vi "test-math-utils.vi"(8 "error in (no error)":errorcluster) -> (0 "error out":errorcluster, 3 "ALL TESTS PASSED":bool)   [LabVIEW 2019]
uses:
  <vilib>/Rock Robotics/WPI/ThirdParty/JAS_Junk/TrajLib/Trajectory_Library.lvlib
panel:
  out "Test 32":bool
  out "Test 31":bool
  out "Test 30":bool
  out "Test 29":bool
  out "Test 28":bool
  out "Test 27":bool
  out "Test 26":bool
  out "Test 25":bool
  out "mod 24":dbl
  out "Test 24":bool
  out "mod 23":dbl
  out "Test 23":bool
  out "mod 22":dbl
  out "Test 22":bool
  out "mod 21":dbl
  out "Test 21":bool
  out "mod 20":dbl
  out "Test 20":bool
  out "mod 19":dbl
  out "Test 19":bool
  out "mod 18":dbl
  out "mod 17":dbl
  out "mod 16":dbl
  out "Test 18":bool
  out "Test 17":bool
  out "Test 16":bool
  out "Test 15":bool
  out "Test 14":bool
  out "Test 13":bool
  out "Test 12":bool
  out "Test 11":bool
  out "Test 10":bool
  out "Test 9":bool
  out "Test 8":bool
  out "Test 7":bool
  out "Test 6":bool
  out "Test 5":bool
  out "Test 4":bool
  out "Test 3":bool
  out "Test 2":bool
  out "Test 1":bool
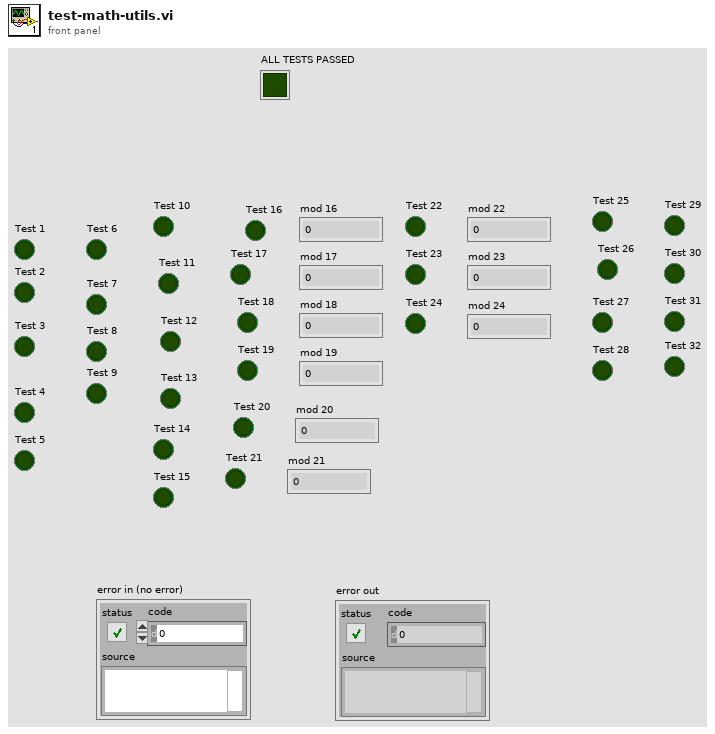
[diagram p1: front panel]
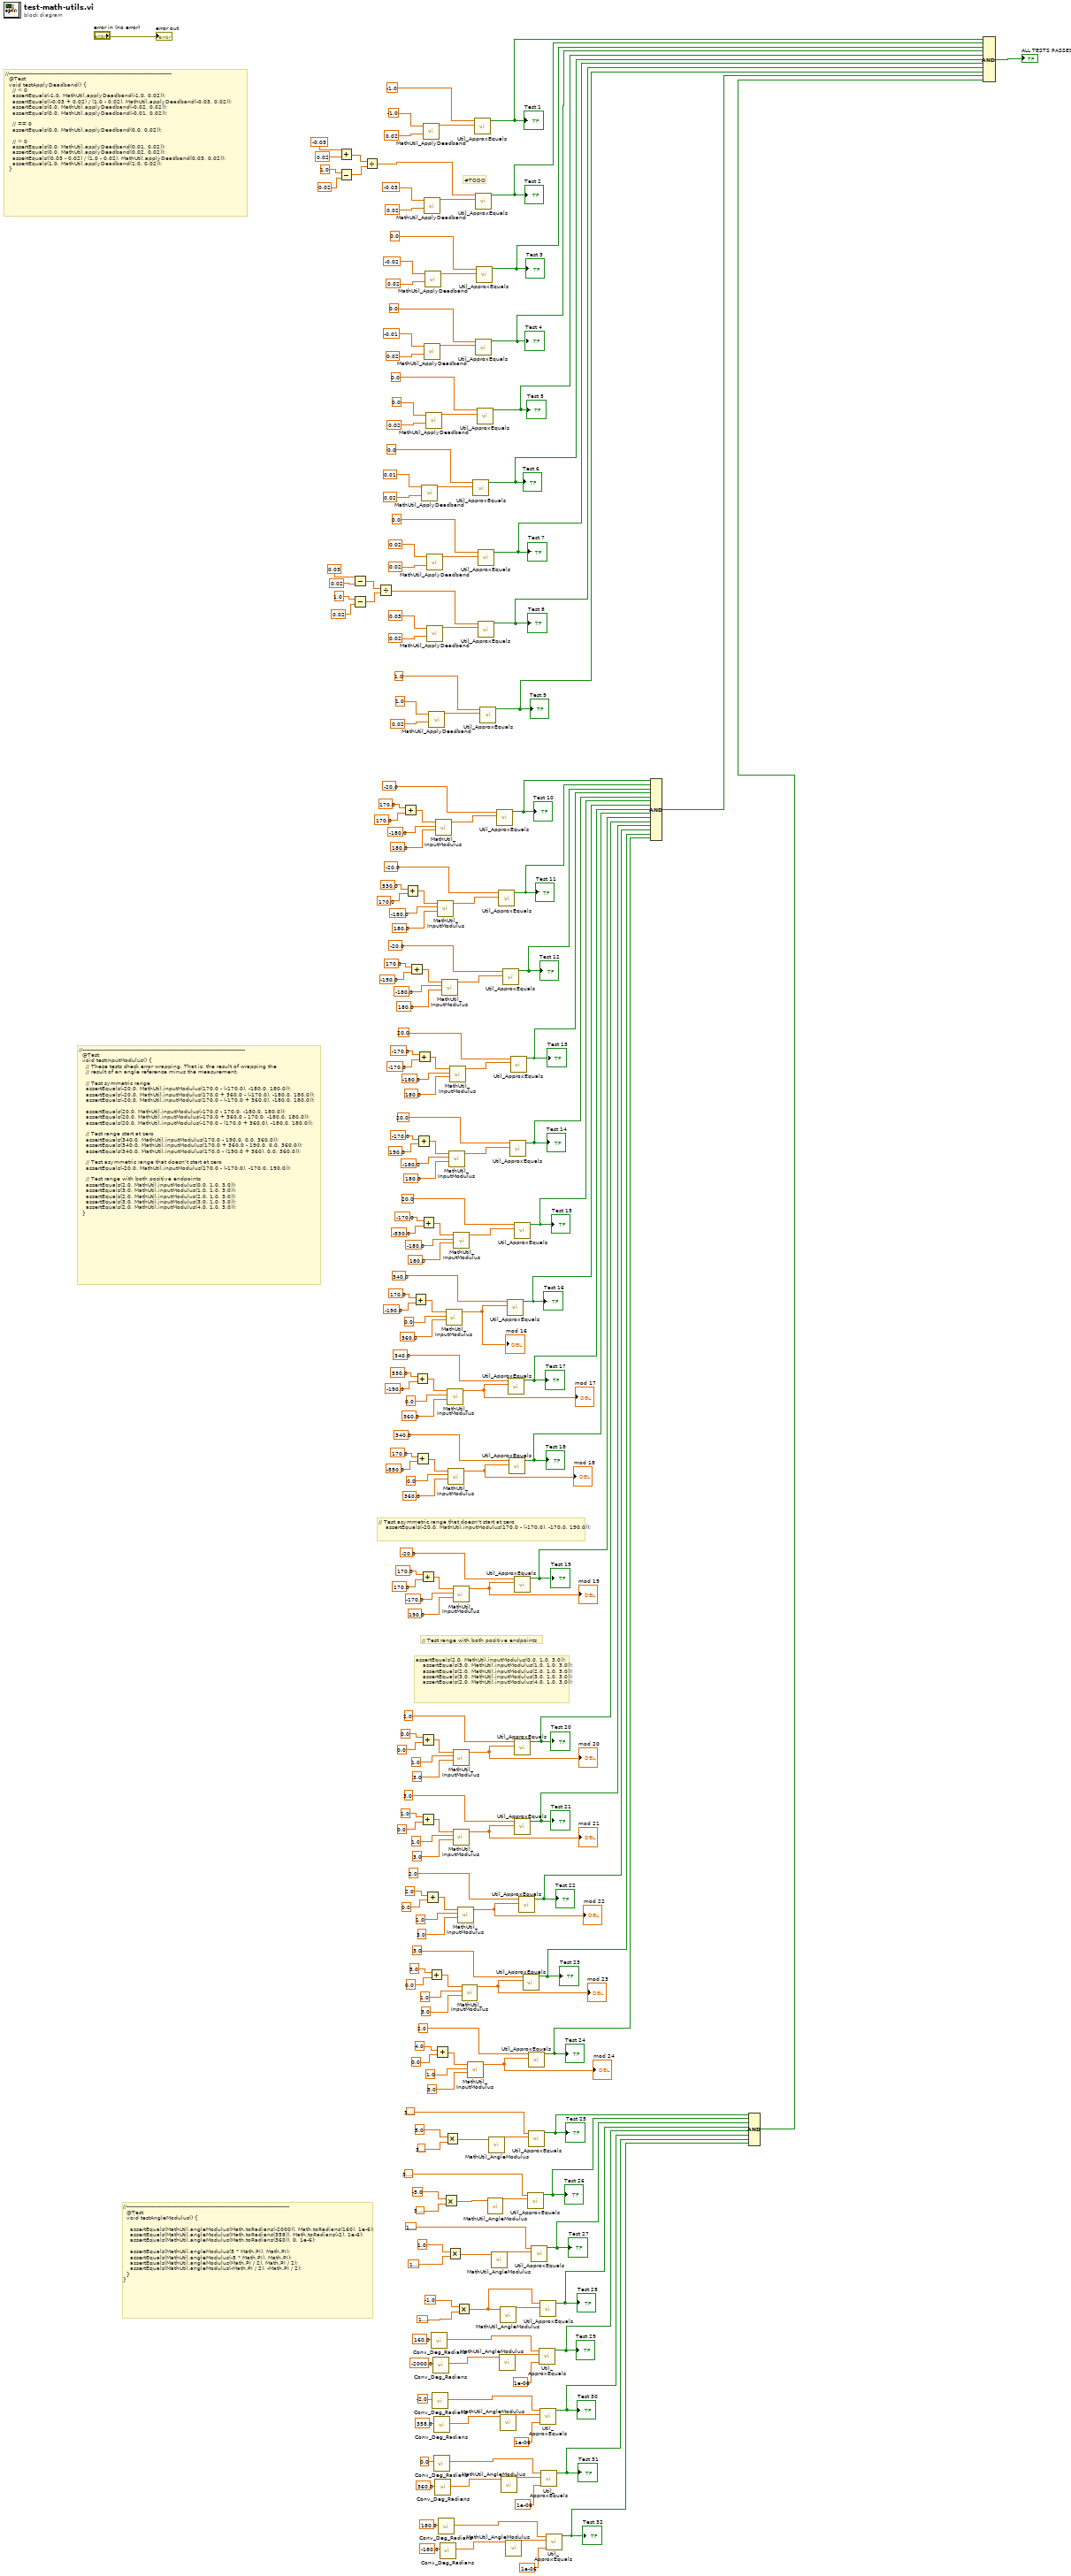
[diagram p0: block diagram]
diagram:
  # "assertEquals(2.0, MathUtil.inputModulus(0.0, 1.0, 3.0));\n    assertEquals(3.0, MathUtil.inputModulus(1.0, 1.0, 3.0));\n    assertEquals(2.0, MathUtil.inputModulus(2.0, 1.0, 3.0));\n    assertEquals(3.0, MathUtil.inputModulus(3.0, 1.0, 3.0));\n    assertEquals(2.0, MathUtil.inputModulus(4.0, 1.0, 3.0));"
  # "// Test range with both positive endpoints"
  # "// Test asymmetric range that doesn't start at zero\n    assertEquals(-20.0, MathUtil.inputModulus(170.0 - (-170.0), -170.0, 190.0));"
  # "#TODO"
  # "//--------------------------------------------------------------------------------------------\n  @Test\n  void testInputModulus() {\n    // These tests check error wrapping. That is, the result of wrapping the\n    // result of an angle reference minus the measurement.\n\n    // Test symmetric range\n    assertEquals(-20.0, MathUtil.inputModulus(170.0 - (-170.0), -180.0, 180.0));\n    assertEquals(-20.0, MathUtil.inputModulus(170.0 + 360.0 - (-170.0), -180.0, 180.0));\n    assertEquals(-20.0, MathUtil.inputModulus(170.0 - (-170.0 + 360.0), -180.0, 180.0));\n\n    assertEquals(20.0, MathUtil.inputModulus(-170.0 - 170.0, -180.0, 180.0));\n    assertEquals(20.0, MathUtil.inputModulus(-170.0 + 360.0 - 170.0, -180.0, 180.0));\n    assertEquals(20.0, MathUtil.inputModulus(-170.0 - (170.0 + 360.0), -180.0, 180.0));\n\n    // Test range start at zero\n    assertEquals(340.0, MathUtil.inputModulus(170.0 - 190.0, 0.0, 360.0));\n    assertEquals(340.0, MathUtil.inputModulus(170.0 + 360.0 - 190.0, 0.0, 360.0));\n    assertEquals(340.0, MathUtil.inputModulus(170.0 - (190.0 + 360), 0.0, 360.0));\n\n    // Test asymmetric range that doesn't start at zero\n    assertEquals(-20.0, MathUtil.inputModulus(170.0 - (-170.0), -170.0, 190.0));\n\n    // Test range with both positive endpoints\n    assertEquals(2.0, MathUtil.inputModulus(0.0, 1.0, 3.0));\n    assertEquals(3.0, MathUtil.inputModulus(1.0, 1.0, 3.0));\n    assertEquals(2.0, MathUtil.inputModulus(2.0, 1.0, 3.0));\n    assertEquals(3.0, MathUtil.inputModulus(3.0, 1.0, 3.0));\n    assertEquals(2.0, MathUtil.inputModulus(4.0, 1.0, 3.0));\n  }"
  # "//--------------------------------------------------------------------------------------------\n  @Test\n  void testApplyDeadband() {\n    // < 0\n    assertEquals(-1.0, MathUtil.applyDeadband(-1.0, 0.02));\n    assertEquals((-0.03 + 0.02) / (1.0 - 0.02), MathUtil.applyDeadband(-0.03, 0.02));\n    assertEquals(0.0, MathUtil.applyDeadband(-0.02, 0.02));\n    assertEquals(0.0, MathUtil.applyDeadband(-0.01, 0.02));\n\n    // == 0\n    assertEquals(0.0, MathUtil.applyDeadband(0.0, 0.02));\n\n    // > 0\n    assertEquals(0.0, MathUtil.applyDeadband(0.01, 0.02));\n    assertEquals(0.0, MathUtil.applyDeadband(0.02, 0.02));\n    assertEquals((0.03 - 0.02) / (1.0 - 0.02), MathUtil.applyDeadband(0.03, 0.02));\n    assertEquals(1.0, MathUtil.applyDeadband(1.0, 0.02));\n  }"
  # "//--------------------------------------------------------------------------------------------\n  @Test\n  void testAngleModulus() {\n\n    assertEquals(MathUtil.angleModulus(Math.toRadians(-2000)), Math.toRadians(160), 1e-6);\n    assertEquals(MathUtil.angleModulus(Math.toRadians(358)), Math.toRadians(-2), 1e-6);\n    assertEquals(MathUtil.angleModulus(Math.toRadians(360)), 0, 1e-6);\n\n    assertEquals(MathUtil.angleModulus(5 * Math.PI), Math.PI);\n    assertEquals(MathUtil.angleModulus(-5 * Math.PI), Math.PI);\n    assertEquals(MathUtil.angleModulus(Math.PI / 2), Math.PI / 2);\n    assertEquals(MathUtil.angleModulus(-Math.PI / 2), -Math.PI / 2);\n  }\n}"
  n1 = Add(x=-0.03, y=0.02) -> (x+y=w187:dbl)
  n2 = Subtract(x=1.0, y=0.02) -> (x-y=w186:dbl)
  n3 = Subtract(x=0.03, y=0.02) -> (x-y=w180:dbl)
  n4 = Subtract(x=1.0, y=0.02) -> (x-y=w179:dbl)
  n5 = Divide(x=w187, y=w186) -> (x/y=w181:dbl)
  n6 = Divide(x=w180, y=w179) -> (x/y=w174:dbl)
  n7 = Add(x=170.0, y=170.0) -> (x+y=w169:dbl)
  n8 = Add(x=530.0, y=170.0) -> (x+y=w162:dbl)
  n9 = Add(x=170.0, y=-190.0) -> (x+y=w155:dbl)
  n10 = Add(x=170.0, y=-190.0) -> (x+y=w127:dbl)
  n11 = Add(x=530.0, y=-190.0) -> (x+y=w120:dbl)
  n12 = Add(x=170.0, y=-550.0) -> (x+y=w113:dbl)
  n13 = Add(x=-170.0, y=190.0) -> (x+y=w141:dbl)
  n14 = Add(x=-170.0, y=-170.0) -> (x+y=w148:dbl)
  n15 = Add(x=170.0, y=170.0) -> (x+y=w106:dbl)
  n16 = Add(x=0.0, y=0.0) -> (x+y=w99:dbl)
  n17 = Add(x=1.0, y=0.0) -> (x+y=w92:dbl)
  n18 = Add(x=-170.0, y=-530.0) -> (x+y=w134:dbl)
  n19 = call <vilib>:"MathUtil_ApplyDeadband.vi"("Deadband"=0.02, "Value"=0.01) -> ("Result"=w211:dbl)  [unwired: 9 in]
  n20 = call <vilib>:"MathUtil_ApplyDeadband.vi"("Deadband"=0.02, "Value"=-1.0) -> ("Result"=w230:dbl)  [unwired: 9 in]
  n21 = call <vilib>:"MathUtil_ApplyDeadband.vi"("Deadband"=0.02, "Value"=-0.03) -> ("Result"=w227:dbl)  [unwired: 9 in]
  n22 = call <vilib>:"MathUtil_ApplyDeadband.vi"("Deadband"=0.02, "Value"=-0.01) -> ("Result"=w219:dbl)  [unwired: 9 in]
  n23 = call <vilib>:"MathUtil_ApplyDeadband.vi"("Deadband"=0.02, "Value"=-0.02) -> ("Result"=w223:dbl)  [unwired: 9 in]
  n24 = Add(x=2.0, y=0.0) -> (x+y=w85:dbl)
  n25 = call <vilib>:"MathUtil_ApplyDeadband.vi"("Deadband"=0.02, "Value"=0.0) -> ("Result"=w215:dbl)  [unwired: 9 in]
  n26 = call <vilib>:"MathUtil_ApplyDeadband.vi"("Deadband"=0.02, "Value"=0.02) -> ("Result"=w207:dbl)  [unwired: 9 in]
  n27 = call <vilib>:"MathUtil_ApplyDeadband.vi"("Deadband"=0.02, "Value"=0.03) -> ("Result"=w204:dbl)  [unwired: 9 in]
  n28 = call <vilib>:"MathUtil_ApplyDeadband.vi"("Deadband"=0.02, "Value"=1.0) -> ("Result"=w200:dbl)  [unwired: 9 in]
  n29 = Add(x=3.0, y=0.0) -> (x+y=w78:dbl)
  n30 = call <vilib>:"Conv_Deg_Radians.vi"("Degress"=160.0) -> ("Radians"=w30:dbl)  [unwired: 10 in]
  n31 = call <vilib>:"Conv_Deg_Radians.vi"("Degress"=-2.0) -> ("Radians"=w24:dbl)  [unwired: 10 in]
  n32 = call <vilib>:"Conv_Deg_Radians.vi"("Degress"=-2000.0) -> ("Radians"=w29:dbl)  [unwired: 10 in]
  n33 = call <vilib>:"Conv_Deg_Radians.vi"("Degress"=0.0) -> ("Radians"=w18:dbl)  [unwired: 10 in]
  n34 = call <vilib>:"Conv_Deg_Radians.vi"("Degress"=358.0) -> ("Radians"=w23:dbl)  [unwired: 10 in]
  n35 = Add(x=4.0, y=0.0) -> (x+y=w71:dbl)
  n36 = call <vilib>:"Conv_Deg_Radians.vi"("Degress"=360.0) -> ("Radians"=w17:dbl)  [unwired: 10 in]
  n37 = call <vilib>:"MathUtil_InputModulus.vi"("Maximum_Input"=180.0, "Minimum_Input"=-180.0, "Input"=w169) -> ("modulus"=w173:dbl)  [unwired: 8 in]
  n38 = call <vilib>:"MathUtil_InputModulus.vi"("Maximum_Input"=180.0, "Minimum_Input"=-180.0, "Input"=w162) -> ("modulus"=w166:dbl)  [unwired: 8 in]
  n39 = call <vilib>:"Conv_Deg_Radians.vi"("Degress"=180.0) -> ("Radians"=w12:dbl)  [unwired: 10 in]
  n40 = call <vilib>:"Conv_Deg_Radians.vi"("Degress"=-180.0) -> ("Radians"=w11:dbl)  [unwired: 10 in]
  n41 = call <vilib>:"MathUtil_InputModulus.vi"("Maximum_Input"=180.0, "Minimum_Input"=-180.0, "Input"=w155) -> ("modulus"=w159:dbl)  [unwired: 8 in]
  n42 = Multiply(x=-5.0, y=3.141592653589793) -> (x*y=w45:dbl)
  n43 = Multiply(x=5.0, y=3.141592653589793) -> (x*y=w50:dbl)
  n44 = call <vilib>:"MathUtil_InputModulus.vi"("Maximum_Input"=360.0, "Minimum_Input"=0.0, "Input"=w127) -> ("modulus"=w131:dbl)  [unwired: 8 in]
  "mod 16" <- w131
  n45 = call <vilib>:"MathUtil_InputModulus.vi"("Maximum_Input"=360.0, "Minimum_Input"=0.0, "Input"=w120) -> ("modulus"=w124:dbl)  [unwired: 8 in]
  "mod 17" <- w124
  n46 = Multiply(x=1.0, y=1.5707963267948966) -> (x*y=w41:dbl)
  n47 = call <vilib>:"MathUtil_InputModulus.vi"("Maximum_Input"=360.0, "Minimum_Input"=0.0, "Input"=w113) -> ("modulus"=w117:dbl)  [unwired: 8 in]
  "mod 18" <- w117
  n48 = call <vilib>:"MathUtil_InputModulus.vi"("Maximum_Input"=180.0, "Minimum_Input"=-180.0, "Input"=w141) -> ("modulus"=w145:dbl)  [unwired: 8 in]
  n49 = call <vilib>:"MathUtil_InputModulus.vi"("Maximum_Input"=180.0, "Minimum_Input"=-180.0, "Input"=w148) -> ("modulus"=w152:dbl)  [unwired: 8 in]
  n50 = call <vilib>:"MathUtil_InputModulus.vi"("Maximum_Input"=190.0, "Minimum_Input"=-170.0, "Input"=w106) -> ("modulus"=w110:dbl)  [unwired: 8 in]
  "mod 19" <- w110
  n51 = call <vilib>:"MathUtil_InputModulus.vi"("Maximum_Input"=3.0, "Minimum_Input"=1.0, "Input"=w99) -> ("modulus"=w103:dbl)  [unwired: 8 in]
  "mod 20" <- w103
  n52 = call <vilib>:"MathUtil_InputModulus.vi"("Maximum_Input"=3.0, "Minimum_Input"=1.0, "Input"=w92) -> ("modulus"=w96:dbl)  [unwired: 8 in]
  "mod 21" <- w96
  n53 = call <vilib>:"MathUtil_InputModulus.vi"("Maximum_Input"=180.0, "Minimum_Input"=-180.0, "Input"=w134) -> ("modulus"=w138:dbl)  [unwired: 8 in]
  n54 = Multiply(x=-1.0, y=1.5707963267948966) -> (x*y=w34:dbl)
  n55 = call <vilib>:"MathUtil_InputModulus.vi"("Maximum_Input"=3.0, "Minimum_Input"=1.0, "Input"=w85) -> ("modulus"=w89:dbl)  [unwired: 8 in]
  "mod 22" <- w89
  n56 = call <vilib>:"MathUtil_InputModulus.vi"("Maximum_Input"=3.0, "Minimum_Input"=1.0, "Input"=w78) -> ("modulus"=w82:dbl)  [unwired: 8 in]
  "mod 23" <- w82
  n57 = call <vilib>:"MathUtil_InputModulus.vi"("Maximum_Input"=3.0, "Minimum_Input"=1.0, "Input"=w71) -> ("modulus"=w75:dbl)  [unwired: 8 in]
  "mod 24" <- w75
  n58 = call <vilib>:"Util_ApproxEquals.vi"("Value 2"=w211, "Value 1"=0.0) -> ("ApproxEquals"=w191:bool)  [unwired: 9 in]
  "Test 6" <- w191
  n59 = call <vilib>:"Util_ApproxEquals.vi"("Value 2"=w230, "Value 1"=-1.0) -> ("ApproxEquals"=w196:bool)  [unwired: 9 in]
  "Test 1" <- w196
  n60 = call <vilib>:"Util_ApproxEquals.vi"("Value 2"=w227, "Value 1"=w181) -> ("ApproxEquals"=w195:bool)  [unwired: 9 in]
  "Test 2" <- w195
  n61 = call <vilib>:"Util_ApproxEquals.vi"("Value 2"=w219, "Value 1"=0.0) -> ("ApproxEquals"=w193:bool)  [unwired: 9 in]
  "Test 4" <- w193
  n62 = call <vilib>:"Util_ApproxEquals.vi"("Value 2"=w223, "Value 1"=0.0) -> ("ApproxEquals"=w194:bool)  [unwired: 9 in]
  "Test 3" <- w194
  n63 = call <vilib>:"Util_ApproxEquals.vi"("Value 2"=w215, "Value 1"=0.0) -> ("ApproxEquals"=w192:bool)  [unwired: 9 in]
  "Test 5" <- w192
  n64 = call <vilib>:"Util_ApproxEquals.vi"("Value 2"=w207, "Value 1"=0.0) -> ("ApproxEquals"=w190:bool)  [unwired: 9 in]
  "Test 7" <- w190
  n65 = call <vilib>:"Util_ApproxEquals.vi"("Value 2"=w204, "Value 1"=w174) -> ("ApproxEquals"=w189:bool)  [unwired: 9 in]
  "Test 8" <- w189
  n66 = call <vilib>:"Util_ApproxEquals.vi"("Value 2"=w200, "Value 1"=1.0) -> ("ApproxEquals"=w188:bool)  [unwired: 9 in]
  "Test 9" <- w188
  n67 = call <vilib>:"MathUtil_AngleModulus.vi"("InputAngle"=w45) -> ("ModulsAngle"=w47:dbl)  [unwired: 10 in]
  n68 = call <vilib>:"MathUtil_AngleModulus.vi"("InputAngle"=w50) -> ("ModulsAngle"=w52:dbl)  [unwired: 10 in]
  n69 = call <vilib>:"MathUtil_AngleModulus.vi"("InputAngle"=w41) -> ("ModulsAngle"=w42:dbl)  [unwired: 10 in]
  n70 = call <vilib>:"Util_ApproxEquals.vi"("Value 2"=w173, "Value 1"=-20.0) -> ("ApproxEquals"=w68:bool)  [unwired: 9 in]
  "Test 10" <- w68
  n71 = call <vilib>:"Util_ApproxEquals.vi"("Value 2"=w166, "Value 1"=-20.0) -> ("ApproxEquals"=w67:bool)  [unwired: 9 in]
  "Test 11" <- w67
  n72 = call <vilib>:"MathUtil_AngleModulus.vi"("InputAngle"=w29) -> ("ModulsAngle"=w33:dbl)  [unwired: 10 in]
  n73 = call <vilib>:"MathUtil_AngleModulus.vi"("InputAngle"=w34) -> ("ModulsAngle"=w37:dbl)  [unwired: 10 in]
  n74 = call <vilib>:"MathUtil_AngleModulus.vi"("InputAngle"=w23) -> ("ModulsAngle"=w27:dbl)  [unwired: 10 in]
  n75 = call <vilib>:"MathUtil_AngleModulus.vi"("InputAngle"=w17) -> ("ModulsAngle"=w21:dbl)  [unwired: 10 in]
  n76 = call <vilib>:"Util_ApproxEquals.vi"("Value 2"=w159, "Value 1"=-20.0) -> ("ApproxEquals"=w66:bool)  [unwired: 9 in]
  "Test 12" <- w66
  n77 = call <vilib>:"MathUtil_AngleModulus.vi"("InputAngle"=w11) -> ("ModulsAngle"=w15:dbl)  [unwired: 10 in]
  n78 = call <vilib>:"Util_ApproxEquals.vi"("Value 2"=w131, "Value 1"=340.0) -> ("ApproxEquals"=w62:bool)  [unwired: 9 in]
  "Test 16" <- w62
  n79 = call <vilib>:"Util_ApproxEquals.vi"("Value 2"=w124, "Value 1"=340.0) -> ("ApproxEquals"=w61:bool)  [unwired: 9 in]
  "Test 17" <- w61
  n80 = call <vilib>:"Util_ApproxEquals.vi"("Value 2"=w117, "Value 1"=340.0) -> ("ApproxEquals"=w60:bool)  [unwired: 9 in]
  "Test 18" <- w60
  n81 = call <vilib>:"Util_ApproxEquals.vi"("Value 2"=w145, "Value 1"=20.0) -> ("ApproxEquals"=w64:bool)  [unwired: 9 in]
  "Test 14" <- w64
  n82 = call <vilib>:"Util_ApproxEquals.vi"("Value 2"=w152, "Value 1"=20.0) -> ("ApproxEquals"=w65:bool)  [unwired: 9 in]
  "Test 13" <- w65
  n83 = call <vilib>:"Util_ApproxEquals.vi"("Value 2"=w110, "Value 1"=-20.0) -> ("ApproxEquals"=w59:bool)  [unwired: 9 in]
  "Test 19" <- w59
  n84 = call <vilib>:"Util_ApproxEquals.vi"("Value 2"=w103, "Value 1"=2.0) -> ("ApproxEquals"=w58:bool)  [unwired: 9 in]
  "Test 20" <- w58
  n85 = call <vilib>:"Util_ApproxEquals.vi"("Value 2"=w96, "Value 1"=3.0) -> ("ApproxEquals"=w57:bool)  [unwired: 9 in]
  "Test 21" <- w57
  n86 = call <vilib>:"Util_ApproxEquals.vi"("Value 2"=w138, "Value 1"=20.0) -> ("ApproxEquals"=w63:bool)  [unwired: 9 in]
  "Test 15" <- w63
  n87 = call <vilib>:"Util_ApproxEquals.vi"("Value 2"=w89, "Value 1"=2.0) -> ("ApproxEquals"=w56:bool)  [unwired: 9 in]
  "Test 22" <- w56
  n88 = call <vilib>:"Util_ApproxEquals.vi"("Value 2"=w82, "Value 1"=3.0) -> ("ApproxEquals"=w55:bool)  [unwired: 9 in]
  "Test 23" <- w55
  n89 = call <vilib>:"Util_ApproxEquals.vi"("Value 2"=w47, "Value 1"=3.141592653589793) -> ("ApproxEquals"=w8:bool)  [unwired: 9 in]
  "Test 26" <- w8
  n90 = call <vilib>:"Util_ApproxEquals.vi"("Value 2"=w75, "Value 1"=2.0) -> ("ApproxEquals"=w54:bool)  [unwired: 9 in]
  "Test 24" <- w54
  n91 = call <vilib>:"Util_ApproxEquals.vi"("Value 2"=w52, "Value 1"=3.141592653589793) -> ("ApproxEquals"=w9:bool)  [unwired: 9 in]
  "Test 25" <- w9
  n92 = call <vilib>:"Util_ApproxEquals.vi"("Value 2"=w42, "Value 1"=1.5707963267948966) -> ("ApproxEquals"=w7:bool)  [unwired: 9 in]
  "Test 27" <- w7
  n93 = call <vilib>:"Util_ApproxEquals.vi"("Tolerance"=1e-06, "Value 2"=w33, "Value 1"=w30) -> ("ApproxEquals"=w5:bool)  [unwired: 8 in]
  "Test 29" <- w5
  n94 = call <vilib>:"Util_ApproxEquals.vi"("Value 2"=w37, "Value 1"=w34) -> ("ApproxEquals"=w6:bool)  [unwired: 9 in]
  "Test 28" <- w6
  n95 = call <vilib>:"Util_ApproxEquals.vi"("Tolerance"=1e-06, "Value 2"=w27, "Value 1"=w24) -> ("ApproxEquals"=w4:bool)  [unwired: 8 in]
  "Test 30" <- w4
  n96 = call <vilib>:"Util_ApproxEquals.vi"("Tolerance"=1e-06, "Value 2"=w21, "Value 1"=w18) -> ("ApproxEquals"=w3:bool)  [unwired: 8 in]
  "Test 31" <- w3
  n97 = call <vilib>:"Util_ApproxEquals.vi"("Tolerance"=1e-06, "Value 2"=w15, "Value 1"=w12) -> ("ApproxEquals"=w2:bool)  [unwired: 8 in]
  "Test 32" <- w2
  n98 = Compound Arithmetic op=AND(w68, w67, w66, w65, w64, w63, w62, w61, w60, w59, w58, w57, w56, w55, w54) -> (w53:bool)
  n99 = Compound Arithmetic op=AND(w9, w8, w7, w6, w5, w4, w3, w2) -> (w1:bool)
  n100 = Compound Arithmetic op=AND(w196, w195, w194, w193, w192, w191, w190, w189, w188, w53, w1) -> (→"ALL TESTS PASSED":bool)
  "error out" <- "error in (no error)"
